vi "Add Component Dependencies.vi"(8 "error in (no error)":errorcluster, 11 "Device Item Ref in":T1 format="%.0x") -> (0 "error out":errorcluster, 2 "component names":string[](array[string]), 3 "Device Ref out":T1 format="%.0x")   [LabVIEW 2017, in "DSF System Explorer.lvlib"]
uses:
  DSF System Explorer.lvlib
  <vilib>/NI Veristand/Custom Device API/Custom Device Item Ref.ctl
  <vilib>/NI Veristand/Custom Device API/Set Item Property (Path).vi
  <vilib>/NI Veristand/Custom Device API/Custom Device API.lvlib
  Shared/DSF Shared.lvlib
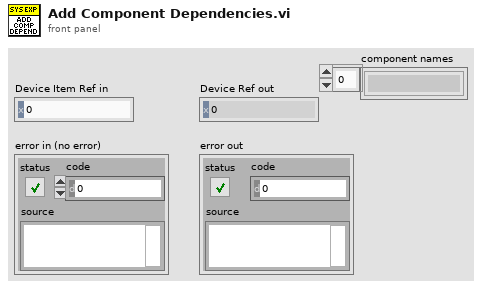
[diagram p1: front panel]
types:
  T1 = typedef "Custom Device API.lvlib/Custom Device Item Ref.ctl" = u64
  T2 = typedef "Custom Device API.lvlib/Custom Device Target Type.ctl" = enum16{"PharLap", "VxWorks", "Windows", "Linux_32_ARM", "Linux_x64"}
  T3 = typedef "Custom Device API.lvlib/Custom Device File Dependency.ctl" = cluster{"Source":T4, "RT Destination":path, "ForceDownload?":bool, "SupportedTarget":T6, "Version":string}
  T4 = typedef "Custom Device API.lvlib/Path Specification.ctl" = cluster{"Path":path, "Type":T5}
  T5 = typedef "Custom Device API.lvlib/Path Type.ctl" = enum16{"Absolute", "To Base", "To Common Data Dir", "To Application Data Dir"}
  T6 = typedef "Custom Device API.lvlib/Custom Device Supported Target.ctl" = enum16{"All", "PharLap", "VxWorks", "Windows", "Linux_32_ARM", "Linux_x64", "PharLap & Windows", "PharLap & VxWorks", "VxWorks & Windows"}
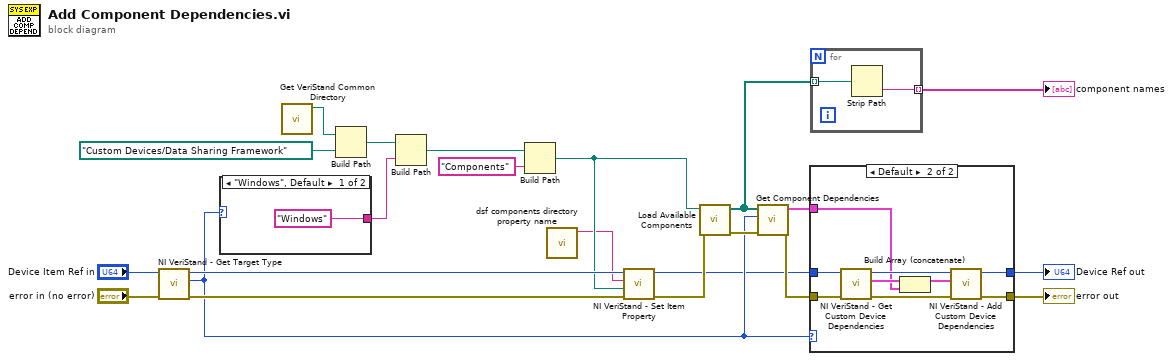
[diagram p0: block diagram]
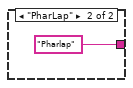
[diagram p3: hidden frame]
diagram:
  n1 = call <vilib>:"NI VeriStand - Get Target Type.vi"("error in (no error)"="error in (no error)", "Item Ref in"="Device Item Ref in") -> ("error out"=w8:errorcluster, "Target Type"=w7:T2, "Item Ref out"=w9:T1)  [unwired: 7 in]
  n2 = case shown="\"Windows\", Default" w7 {
    tunnel: ["Windows" "Pharlap"] -> w12
    frame "Windows", Default {
    }
    frame "PharLap" {
    }
  }
  n3 = call "Get VeriStand Common Directory.vi"() -> ("common directory"=w15:path)  [unwired: 11 in]
  n4 = Build Path(base path=w15, name or relative path=path "Custom Devices/Data Sharing Framework") -> (appended path=w17:path)
  n5 = Build Path(base path=w17, name or relative path=w12) -> (appended path=w13:path)
  n6 = Build Path(base path=w13, name or relative path="Components") -> (appended path=w4:path)
  n7 = call "dsf components directory property name.vi"() -> ("components directory property name"=w3:string)  [unwired: 11 in]
  n8 = call-poly <vilib>:"NI VeriStand - Set Item Property.vi"("error in (no error)"=w8, "Value"=w4, "Property Name"=w3, "Item Ref in"=w9) -> ("error out"=w6:errorcluster, "Item Ref out"=w5:T1)  [unwired: 5 in, 1 out]
  n9 = call "Load Available Components.vi"("error in (no error)"=w6, "components directory"=w4) -> ("error out"=w18:errorcluster, "component paths"=w11:path[])  [unwired: 8 in]
  n10 = call "Get Component Dependencies.vi"("error in (no error)"=w18, "Target Type"=w7, "component paths"=w11) -> ("error out"=w20:errorcluster, "component dependencies"=w19:T3[])  [unwired: 7 in]
  n11 = case shown="Default" w7 {
    tunnel: w19 -> [_ w28]
    tunnel: w20 -> [w26 w34]
    tunnel: w5 -> [w25 w35]
    tunnel: [w26 w29] -> w21
    tunnel: [w25 w27] -> w22
    frame "Windows" {
      # "Don't add dependencies for Windows."
    }
    frame Default {
      n12 = call <vilib>:"NI VeriStand - Get Custom Device Dependencies.vi"("error in (no error)"=w34, "Device Ref in"=w35) -> ("error out"=w32:errorcluster, "Dependencies"=w33:T3[], "Device Ref out"=w30:T1)  [unwired: 7 in]
      n13 = Build Array (concatenate)(w33, w28) -> (w31:T3[])
      n14 = call <vilib>:"NI VeriStand - Add Custom Device Dependencies.vi"("error in (no error)"=w32, "Dependencies"=w31, "Device Ref in"=w30) -> ("error out"=w29:errorcluster, "Device Ref out"=w27:T1)  [unwired: 7 in]
    }
  }
  "Device Ref out" <- w22
  "error out" <- w21
  n15 = for {
    tunnel: w11 -> [w37] mode=indexing
    tunnel: [w36] -> w10 mode=indexing
    n16 = Strip Path(path=w37) -> (name=w36:string)  [unwired: 1 out]
  }
  "component names" <- w10
